vi "英维克系统参数解析.vi"(11 "系统参数输入":u16[](array[numeric])) -> (3 "系统参数":T1)   [LabVIEW 2016, in "环境动力监测库.lvlib" / "空调库.lvlib"]
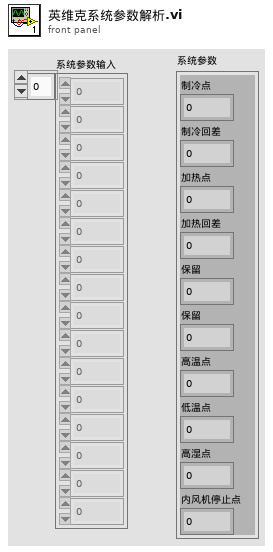
[diagram p1: front panel]
types:
  T1 = cluster{"制冷点":u16, "制冷回差":u16, "加热点":u16, "加热回差":u16, "保留":u16, "保留":u16, "高温点":u16, "低温点":u16, "高湿点":u16, "内风机停止点":u16}
  T2 = cluster{u16, u16, u16, u16, u16, u16, u16, u16, u16, u16}
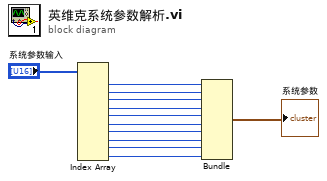
[diagram p0: block diagram]
diagram:
  n1 = Index Array(array="系统参数输入") -> (element #1=w11:u16, element #2=w10:u16, element #3=w9:u16, element #4=w8:u16, element #5=w7:u16, element #6=w6:u16, element #7=w5:u16, element #8=w4:u16, element #9=w3:u16, element #10=w2:u16)  [unwired: 10 in]
  n2 = Bundle(w11, w10, w9, w8, w7, w6, w5, w4, w3, w2) -> (→"系统参数":T2)  [unwired: 1 in]
